vi "Module Loop.vi"(8 "error in (no error)":errorcluster, 11 "Historian Logger in":refnum<class "Historian Logger.lvclass">) -> (0 "error out":errorcluster, 3 "Historian Logger out":refnum<class "Historian Logger.lvclass">)   [LabVIEW 2020, in "VolatusHistorian.lvlib" / "Historian Logger.lvclass"]
uses:
  Historian Logger.lvclass
  C:/dev/lv20CE/relink/lv-volatus/Volatus/Module/Module.lvclass
  Volatus/Module/Module.lvclass
  Volatus/Module/Module.lvclass/Module.ctl
  Historian Logger.lvclass/Historian Logger.ctl
  Logger Status Value/Logger Status Value.lvclass/Logger Status Value.ctl
  VolatusData/Logger Ready.ctl
  VolatusData/Logger Started.ctl
  VolatusData/Logger Stopped.ctl
  <vilib>/Utility/error.llb/Error Cluster From Error Code.vi
  lv-promises/Promises/Promise/Promise.lvclass
  Logger Status Value/Logger Status Value.lvclass
  Volatus/MessageQ/MessageQ.lvclass
  VolatusData/VolatusData.lvlib
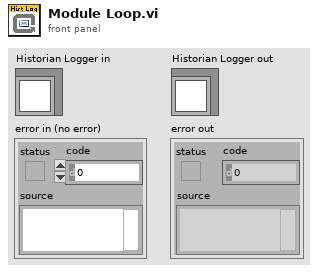
[diagram p1: front panel]
types:
  T1 = enum32{"Invalid", "Standard", "Closed", "Hidden", "Minimized", "Maximized"}
  T2 = typedef "VolatusData.lvlib/Logger Ready.ctl" = cluster{"ID":string}
  T3 = typedef "VolatusData.lvlib/Logger Started.ctl" = cluster{"ID":string}
  T4 = typedef "VolatusData.lvlib/Logger Stopped.ctl" = cluster{"ID":string}
  T5 = typedef "VolatusHistorian.lvlib/Logger Status.ctl" = cluster{"Count":i32, "Log Time":dbl}
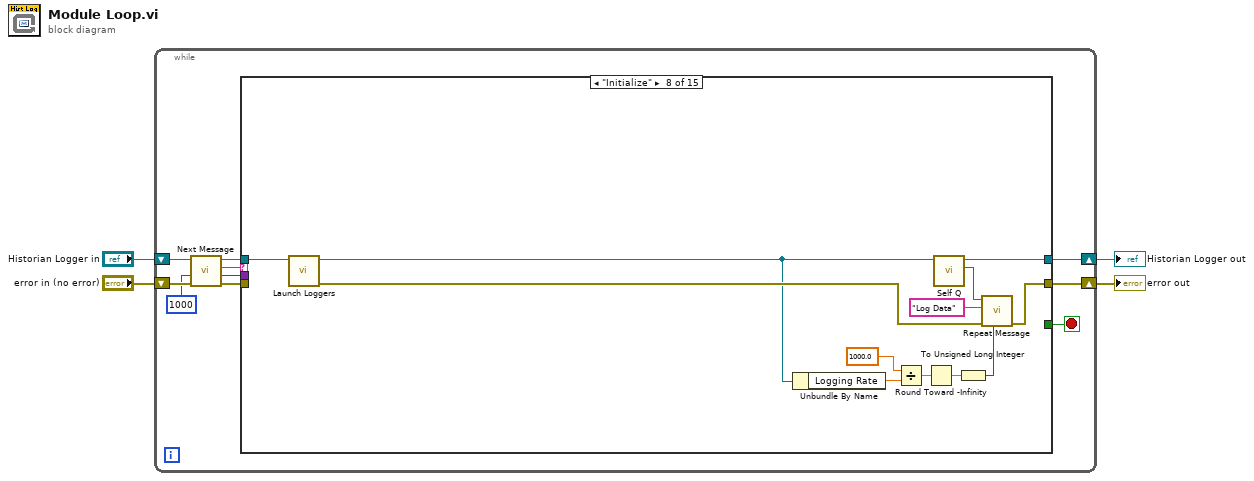
[diagram p0: block diagram]
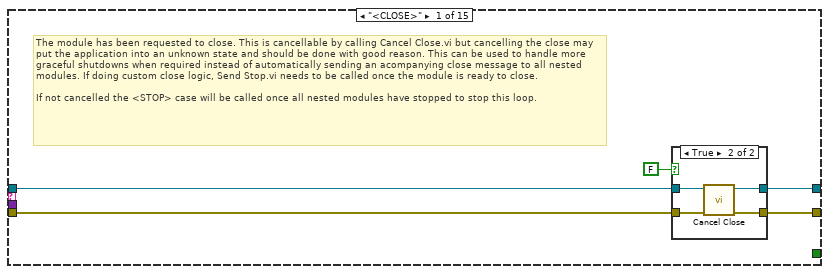
[diagram p2: hidden frame]
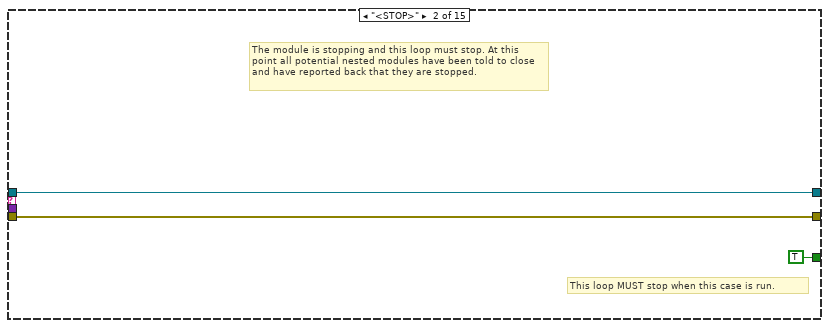
[diagram p4: hidden frame]
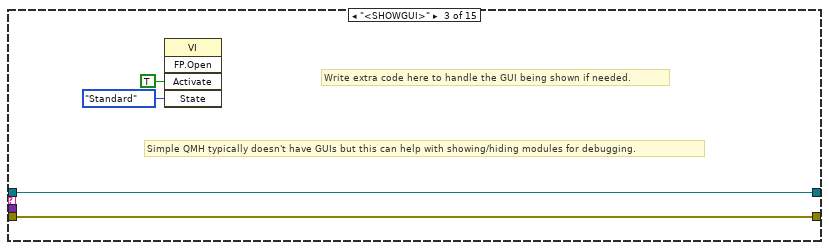
[diagram p5: hidden frame]
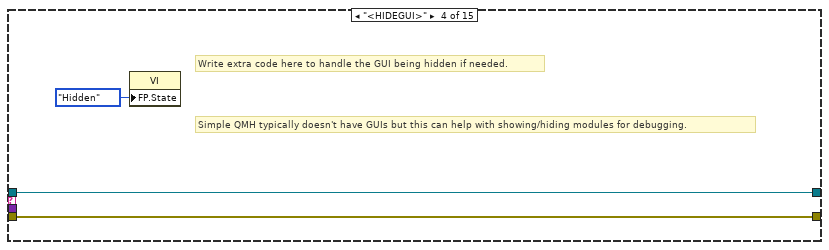
[diagram p6: hidden frame]
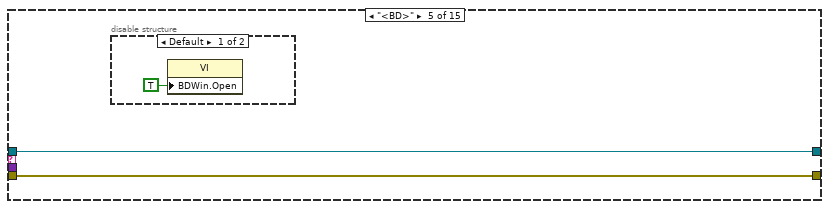
[diagram p7: hidden frame]
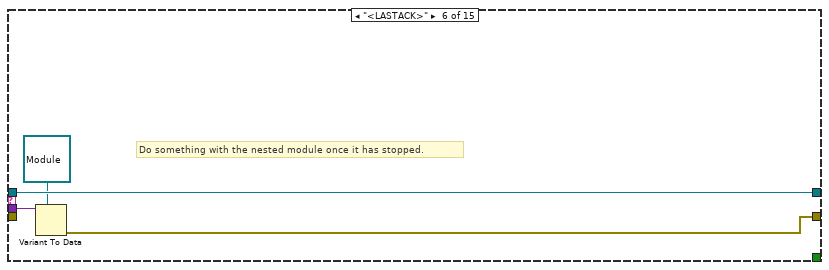
[diagram p9: hidden frame]
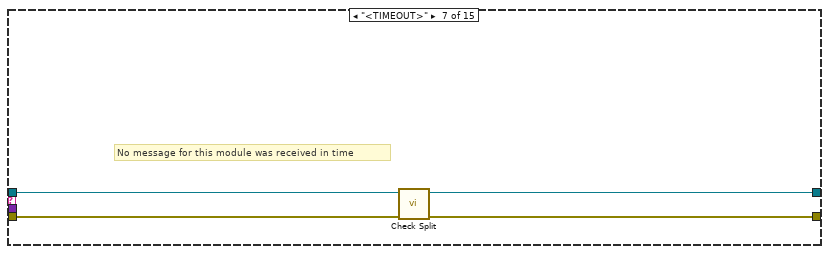
[diagram p10: hidden frame]
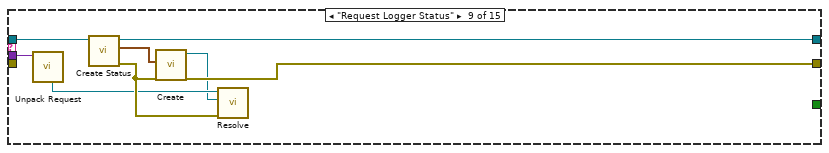
[diagram p11: hidden frame]
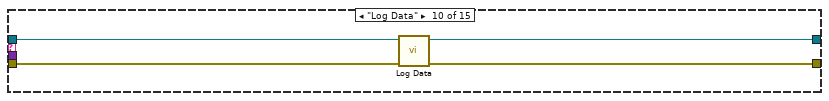
[diagram p12: hidden frame]
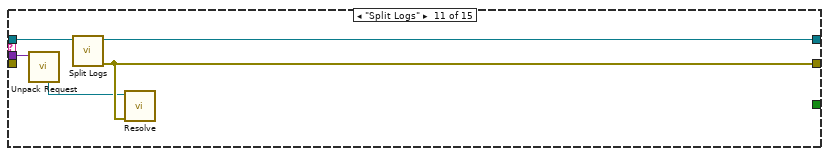
[diagram p13: hidden frame]
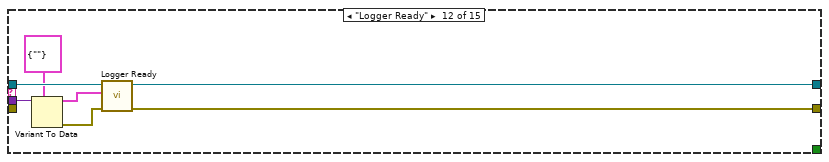
[diagram p14: hidden frame]
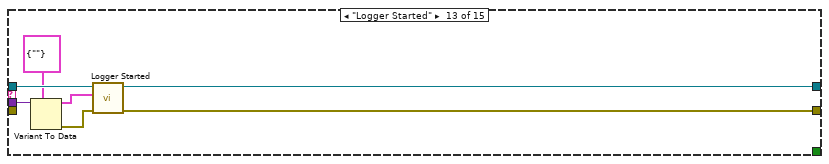
[diagram p15: hidden frame]
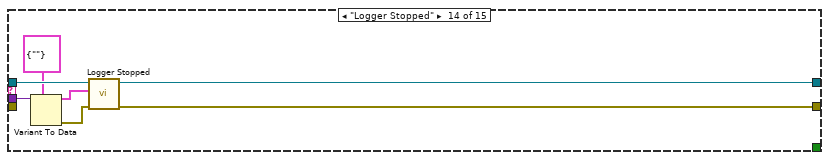
[diagram p16: hidden frame]
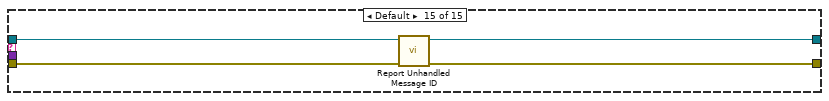
[diagram p17: hidden frame]
diagram:
  n1 = while {
    shift-right: [w9] -> w2
    shift-left: "Historian Logger in" -> [w14]
    shift-right: [w8] -> w1
    shift-left: "error in (no error)" -> [w13]
    stop <- w7 stop-if-true
    n2 = call "Next Message.vi"("error in (no error)"=w13, "Timeout ms (-1)"=1000, "Module in"=w14) -> ("error out"=w12:errorcluster, "Data"=w6:variant, "ID"=w11:string, "Module out"=w10:refnum<class "Historian Logger.lvclass">)  [unwired: 5 in]
    n3 = case shown="\"Initialize\"" w11 {
      tunnel: w12 -> [w19 w27 w31 w34 w36 _ w46 _ _ w69 _ _ _ _ w99]
      tunnel: w10 -> [w17 w28 w32 w35 w37 w42 w44 w54 w64 w67 w74 w81 w88 w95 w97]
      tunnel: [w16 w28 w32 w35 w37 w42 w43 w57 w60 w66 w73 w78 w85 w92 w96] -> w9
      tunnel: [w18 w27 w31 w34 w36 w39 w45 w48 w65 w68 w71 w75 w82 w89 w98] -> w8
      tunnel: [_ TRUE _ _ _ _ _ _ _ _ _ _ _ _ _] -> w7
      tunnel: w6 -> [_ _ _ _ _ w41 _ _ w63 _ w72 w80 w87 w94 _]
      frame "<CLOSE>" {
        # "The module has been requested to close. This is cancellable by calling Cancel Close.vi but cancelling the close may put the application into an unknown state and should be done with good reason. This can be used to handle more graceful shutdowns when required instead of automatically sending an acompanying close message to all nested modules. If doing custom close logic, Send Stop.vi needs to be called once the module is ready to close.\n\nIf not cancelled the <STOP> case will be called once all nested modules have stopped to stop this loop."
        n4 = case shown="True" FALSE {
          tunnel: w19 -> [w20 w25]
          tunnel: [w20 w24] -> w18
          tunnel: w17 -> [w21 w23]
          tunnel: [w21 w22] -> w16
          frame False {
          }
          frame True {
            n5 = call "Cancel Close.vi"("error in (no error)"=w25, "Module in"=w23) -> ("error out"=w24:errorcluster, "Module out"=w22:refnum<class "Historian Logger.lvclass">)  [unwired: 8 in]
          }
        }
      }
      frame "<STOP>" {
        # "This loop MUST stop when this case is run."
        # "The module is stopping and this loop must stop. At this point all potential nested modules have been told to close and have reported back that they are stopped."
      }
      frame "<SHOWGUI>" {
        # "Simple QMH typically doesn't have GUIs but this can help with showing/hiding modules for debugging."
        # "Write extra code here to handle the GUI being shown if needed."
        n6 = invoke class="VI" method="FP.Open"("Activate"=TRUE ("Activate?"), "State"=T1."Standard") -> ()  [unwired: 3 in, 5 out]
      }
      frame "<HIDEGUI>" {
        # "Simple QMH typically doesn't have GUIs but this can help with showing/hiding modules for debugging."
        # "Write extra code here to handle the GUI being hidden if needed."
        n7 = property class="VI"("FP.State"=T1."Hidden" ("Front Panel Window:State")) -> ()  [unwired: 2 in, 2 out]
      }
      frame "<BD>" {
        n8 = disable-structure shown="Default" {
          frame condition #0 (active) {
            n9 = property class="VI"("BDWin.Open"=TRUE ("Block Diagram Window:Open")) -> ()  [unwired: 2 in, 2 out]
          }
          frame condition #1 {
          }
        }
      }
      frame "<LASTACK>" {
        # "Do something with the nested module once it has stopped."
        n10 = Variant To Data(type=refnum<class "Module.lvclass"> refnum ("Volatus:Module"), Variant=w41) -> (error out=w39:errorcluster)  [unwired: 1 in, 1 out]
      }
      frame "<TIMEOUT>" {
        # "No message for this module was received in time"
        n11 = call "Check Split.vi"("error in (no error)"=w46, "Historian Logger in"=w44) -> ("error out"=w45:errorcluster, "Historian Logger out"=w43:refnum<class "Historian Logger.lvclass">)  [unwired: 8 in]
      }
      frame "Initialize" {
        n12 = call "Launch Loggers.vi"("Historian Logger in"=w54) -> ("error out"=w58:errorcluster, "Historian Logger out"=w47:refnum<class "Historian Logger.lvclass">)  [unwired: 9 in]
        n13 = Unbundle By Name(w47) -> ("Logging Rate"=w52:dbl)
        n14 = Divide(x=1000.0, y=w52) -> (x/y=w51:dbl)
        n15 = Round Toward -Infinity(1:w51) -> (0:w50:dbl)
        n16 = call "Self Q.vi"("Module in"=w47) -> ("Self Q"=w56:refnum<class "MessageQ.lvclass">, "Module out"=w57:refnum<class "Historian Logger.lvclass">)  [unwired: 9 in]
        n17 = To Unsigned Long Integer(number=w50) -> (unsigned 32bit integer=w49:u32)
        n18 = call "Repeat Message.vi"("Period ms"=w49, "error in (no error)"=w58, "ID"="Log Data", "MessageQ in"=w56) -> ("error out"=w48:errorcluster)  [unwired: 5 in, 2 out]
      }
      frame "Request Logger Status" {
        n19 = call "Unpack Request.vi"("Request Data"=w63) -> ("Promise"=w62:refnum<class "Promise.lvclass">)  [unwired: 8 in, 2 out]
        n20 = call "Create Status.vi"("Historian Logger in"=w64) -> ("error out"=w65:errorcluster, "Logger Status"=w59:T5, "Historian Logger out"=w60:refnum<class "Historian Logger.lvclass">)  [unwired: 8 in]
        n21 = call "Create.vi"("Logger Status"=w59) -> ("Logger Status Value out"=w61:refnum<class "Logger Status Value.lvclass">)  [unwired: 10 in]
        n22 = call "Resolve.vi"("error in (no error)"=w65, "Result (None)"=w61, "Promise in"=w62) -> ()  [unwired: 7 in, 2 out]
      }
      frame "Log Data" {
        n23 = call "Log Data.vi"("error in (no error)"=w69, "Historian Logger in"=w67) -> ("error out"=w68:errorcluster, "Historian Logger out"=w66:refnum<class "Historian Logger.lvclass">)  [unwired: 8 in]
      }
      frame "Split Logs" {
        n24 = call "Unpack Request.vi"("Request Data"=w72) -> ("Promise"=w70:refnum<class "Promise.lvclass">)  [unwired: 8 in, 2 out]
        n25 = call "Split Logs.vi"("Historian Logger in"=w74) -> ("error out"=w71:errorcluster, "Historian Logger out"=w73:refnum<class "Historian Logger.lvclass">)  [unwired: 9 in]
        n26 = call "Resolve.vi"("error in (no error)"=w71, "Promise in"=w70) -> ()  [unwired: 8 in, 2 out]
      }
      frame "Logger Ready" {
        n27 = Variant To Data(type=T2 {"ID"=""} ("Logger Ready"), Variant=w80) -> (data=w77:T2, error out=w76:errorcluster)  [unwired: 1 in]
        n28 = call "Logger Ready.vi"("error in (no error)"=w76, "Logger Ready"=w77, "Historian Logger in"=w81) -> ("error out"=w75:errorcluster, "Historian Logger out"=w78:refnum<class "Historian Logger.lvclass">)  [unwired: 7 in]
      }
      frame "Logger Started" {
        n29 = Variant To Data(type=T3 {"ID"=""} ("Logger Started"), Variant=w87) -> (data=w84:T3, error out=w83:errorcluster)  [unwired: 1 in]
        n30 = call "Logger Started.vi"("error in (no error)"=w83, "Logger Started"=w84, "Historian Logger in"=w88) -> ("error out"=w82:errorcluster, "Historian Logger out"=w85:refnum<class "Historian Logger.lvclass">)  [unwired: 7 in]
      }
      frame "Logger Stopped" {
        n31 = Variant To Data(type=T4 {"ID"=""} ("Logger Stopped"), Variant=w94) -> (data=w91:T4, error out=w90:errorcluster)  [unwired: 1 in]
        n32 = call "Logger Stopped.vi"("error in (no error)"=w90, "Logger Stopped"=w91, "Historian Logger in"=w95) -> ("error out"=w89:errorcluster, "Historian Logger out"=w92:refnum<class "Historian Logger.lvclass">)  [unwired: 7 in]
      }
      frame Default {
        n33 = call "Report Unhandled Message ID.vi"("error in (no error)"=w99, "Module in"=w97) -> ("error out"=w98:errorcluster, "Module out"=w96:refnum<class "Historian Logger.lvclass">)  [unwired: 8 in]
      }
    }
  }
  "error out" <- w1
  "Historian Logger out" <- w2
